vi "frw_array2edf.vi"(6 "channel names":string[](array[string]), 8 "error in":errorcluster, 9 "fs":dbl, 10 "2D array":dbl[][](array[numeric]), 11 "file path":path) -> (0 "error out":errorcluster, 3 "path out":path)   [LabVIEW 2013]
uses:
  <vilib>/addons/Biomedical/File IO/subVIs/biosignal channel property.ctl
  <vilib>/addons/Biomedical/NI_BMTK_FileIO.lvlib
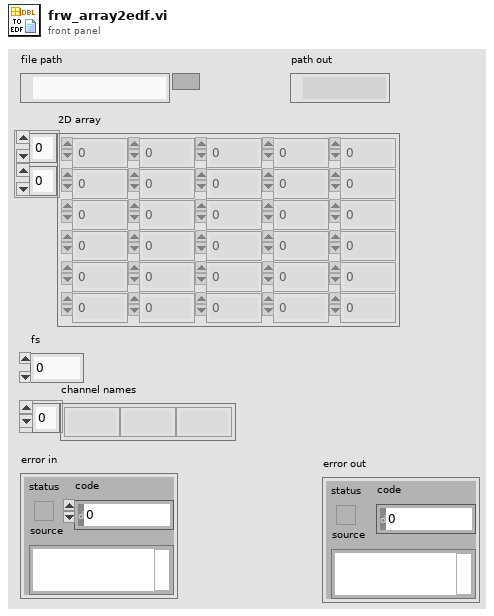
[diagram p1: front panel]
types:
  T1 = typedef "NI_BMTK_FileIO.lvlib/biosignal channel property.ctl" = cluster{"name":string, "unit":string, "description":string, "sampling rate":dbl}
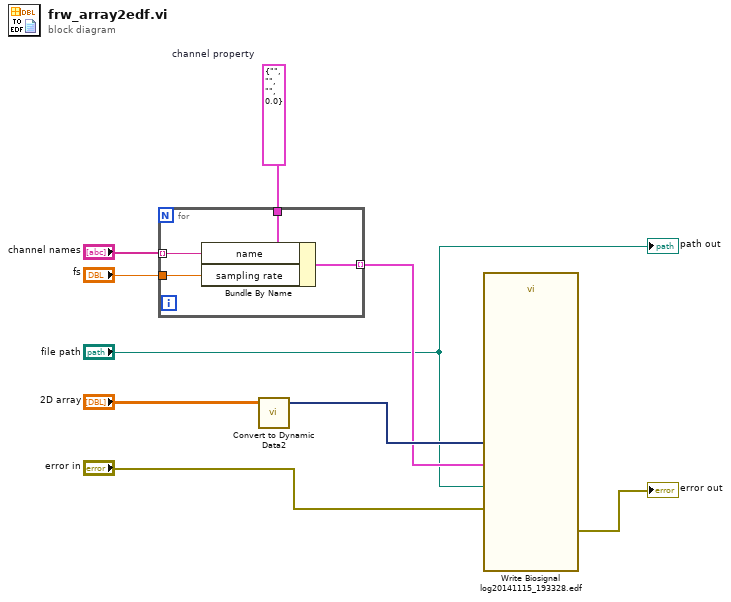
[diagram p0: block diagram]
diagram:
  w4 = T1 {"name"="", "unit"="", "description"="", "sampling rate"=0.0}  # channel property
  n1 = for {
    tunnel: w4 -> [w13]
    tunnel: [w12] -> w7 mode=indexing
    tunnel: "channel names" -> [w11] mode=indexing
    tunnel: "fs" -> [w10]
    n2 = Bundle By Name(cluster=w13, "name"=w11, "sampling rate"=w10) -> (w12:T1)
  }
  n3 = call "Convert to Dynamic Data2"("2D Array"="2D array") -> ("Dynamic Data Type"=w8:dynamicdata)  [unwired: 3 in]
  n4 = call "Write Biosignal\nlog20141115_193328.edf"("file path"="file path", "error in (no error)"="error in", "channel properties"=w7, "biosignals"=w8) -> ("error out"=→"error out":errorcluster)  [unwired: 7 in]
  "path out" <- "file path"
